vi "triangle wave.vi"() -> ()   [LabVIEW 2014]
panel:
  in  "Transfer and Run Date Folder After Experiment":bool
  in  "SSH user name":string
  in  "SSH password":string
  in  "Wait before recording (s)":dbl
  in  "Tags":string
  in  "Start Recording":bool
  in  "Max Power (uW/mm^2)":dbl
  in  "Min Power (uW/mm^2)":dbl
  in  "Frames":i32
  in  "period (frames)":dbl
  in  "Initial Power (uW/mm^2)":dbl
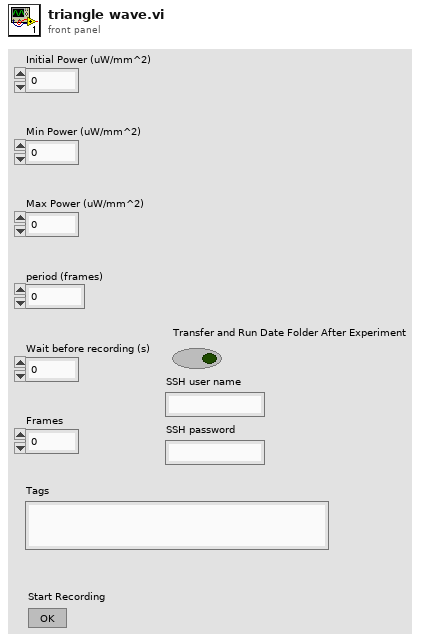
[diagram p1: front panel]
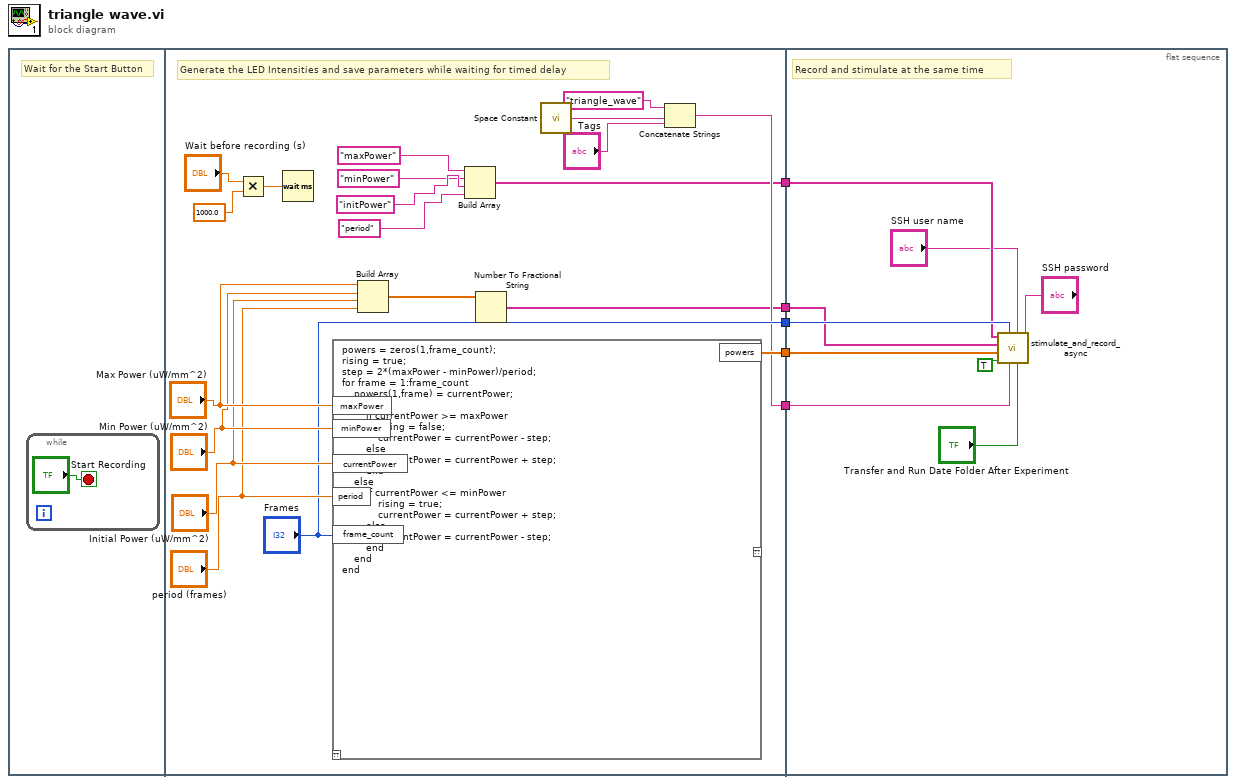
[diagram p0: block diagram]
diagram:
  n1 = flat-sequence {
    tunnel: [w26] -> w5
    tunnel: ["Frames"] -> w4
    tunnel: [w13] -> w3
    tunnel: [w11] -> w2
    tunnel: [w10] -> w1
    tunnel: w5 -> [w32]
    tunnel: w4 -> [w35]
    tunnel: w3 -> [w34]
    tunnel: w2 -> [w31]
    tunnel: w1 -> [w30]
    frame #0 {
      # "Wait for the Start Button"
      n2 = while {
        stop <- "Start Recording" stop-if-true
      }
    }
    frame #1 {
      # "Generate the LED Intensities and save parameters while waiting for timed delay"
      n3 = Multiply(x="Wait before recording (s)", y=1000.0) -> (x*y=w8:dbl)
      n4 = Wait (ms)(milliseconds to wait=w8) -> ()  [unwired: 1 out]
      n5 = script code="powers = zeros(1,frame_count);\nrising = true;\nstep = 2*(maxPower - minPower)/period;\nfor frame = 1:frame_count\n    powers(1,frame) = currentPower;\n    if rising\n        if currentPower >= maxPower\n            rising = false;\n            currentPower = currentPower - step;\n        else\n            currentPower = currentPower + step;\n        end\n    else\n        if currentPower <= minPower\n            rising = true;\n            currentPower = currentPower + step;\n        else\n            currentPower = currentPower - step;\n        end\n    end\nend"("currentPower"="Initial Power (uW/mm^2)", "frame_count"="Frames", "period"="period (frames)", "minPower"="Min Power (uW/mm^2)", "maxPower"="Max Power (uW/mm^2)") -> ("powers"=w26:dbl[])  [unwired: 1 in, 1 out]
      n6 = Build Array("Max Power (uW/mm^2)", "Min Power (uW/mm^2)", "Initial Power (uW/mm^2)", "period (frames)") -> (w12:dbl[])
      n7 = Build Array("maxPower", "minPower", "initPower", "period") -> (w10:string[])
      n8 = Number To Fractional String(number=w12) -> (F-format string=w11:string[])  [unwired: 3 in]
      n9 = call <vilib>:"Space Constant.vi"() -> ("String"=w24:string)
      n10 = Concatenate Strings("triangle_wave", w24, "Tags") -> (w13:string)
    }
    frame #2 {
      # "Record and stimulate at the same time"
      n11 = call "stimulate_and_record_async.vi"("SSH password"="SSH password", "Transfer and Run Date Folder After Experiment"="Transfer and Run Date Folder After Experiment", "SSH user name"="SSH user name", "Tags"=w34, "Frames"=w35, "Convert Power to Voltage"=TRUE, "voltages/power"=w32, "parameters"=w31, "parameters headers"=w30) -> ()  [unwired: 3 in]
    }
  }
